vi "comm close.vi"(4 "error in (no error)":errorcluster, 7 "Comm Handle":u64) -> (0 "error out":errorcluster)   [LabVIEW 2021, in "lvserial.lvlib"]
doc: "Closes the handle (may be the case that only the duplicate of a handle will be closed)."
uses:
  lvserial.lvlib
  lvserial.dll
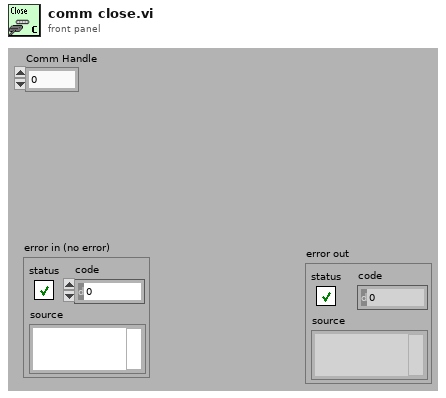
[diagram p1: front panel]
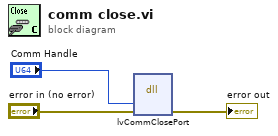
[diagram p0: block diagram]
diagram:
  n1 = dll-call lib="lvserial.dll" fn="lvCommClosePort"("hComm"="Comm Handle", "error"="error in (no error)") -> ("error"=→"error out":errorcluster)  [unwired: 4 in, 3 out]
